vi "Send Example.vi"(0 "Input Data":T1 {"Command" format="%02x"; "Destination" format="%02x"; "Source" format="%02x"}, 1 "Retry Count":u32=3, 11 "Error In":errorcluster) -> (15 "Error Out":errorcluster)   [LabVIEW 2014]
doc: "This standalone VI sends a GEA2 message to the destination you specify."
uses:
  type defs/Data In.ctl
  library/GEA2_Toolkit.lvlib
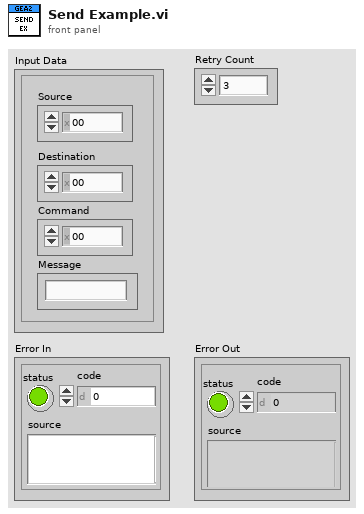
[diagram p1: front panel]
types:
  T1 = typedef "GEA2_Toolkit.lvlib/Data In.ctl" = cluster{"Source":u8, "Destination":u8, "Command":u8, "Message":string}
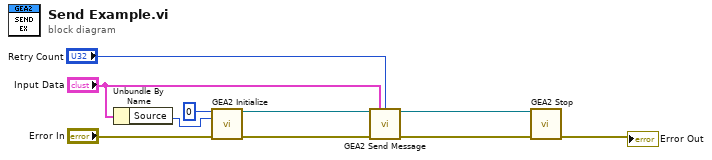
[diagram p0: block diagram]
diagram:
  n1 = Unbundle By Name("Input Data") -> ("Source"=w1:u8)
  n2 = call "GEA2 Initialize.vi"("Board Index"=0, "Source Address"=w1, "error in"="Error In") -> ("GEA2 Reference Out"=w10:refnum<k24>, "error out"=w7:errorcluster)  [unwired: 10 in, 1 out]
  n3 = call "GEA2 Send Message.vi"("GEA2 Reference In"=w10, "Input Data"="Input Data", "Retry Count"="Retry Count", "Error In"=w7) -> ("GEA2 Reference Out"=w9:refnum<k24>, "Error Out"=w8:errorcluster)  [unwired: 10 in]
  n4 = call "GEA2 Stop.vi"("GEA2 Reference In"=w9, "Error In"=w8) -> ("Error Out"=→"Error Out":errorcluster)  [unwired: 13 in]
